vi "IRMouseAttempt.vi"() -> ()   [LabVIEW 2009]
uses:
  wiimotestate.ctl
  wiimoteState(IR).ctl
  C:/Documents and Settings/pbooth/My Documents/labWOOOO/WiimoteLib.dll
  User32.dll
panel:
  out "IR Camera Targets":picture
  out "Cluster":cluster{"Wiimote State":T1, "IRState":T2} {"IRState"."Mode" items=["Off"=0, "Basic"=1, "Extended"=3, "Full"=5]}
  in  "stop":bool
  out "error out":errorcluster
  # "Establish a Bluetooth link with your Wiimote prior to executing this VI.\n\nRequires the Wiimote Managed Library WiimoteLib Ver 1.7\navailable from http://www.codeplex.com/WiimoteLib\nSam Shearman"
  # "Accelerometers"
  # "Buttons"
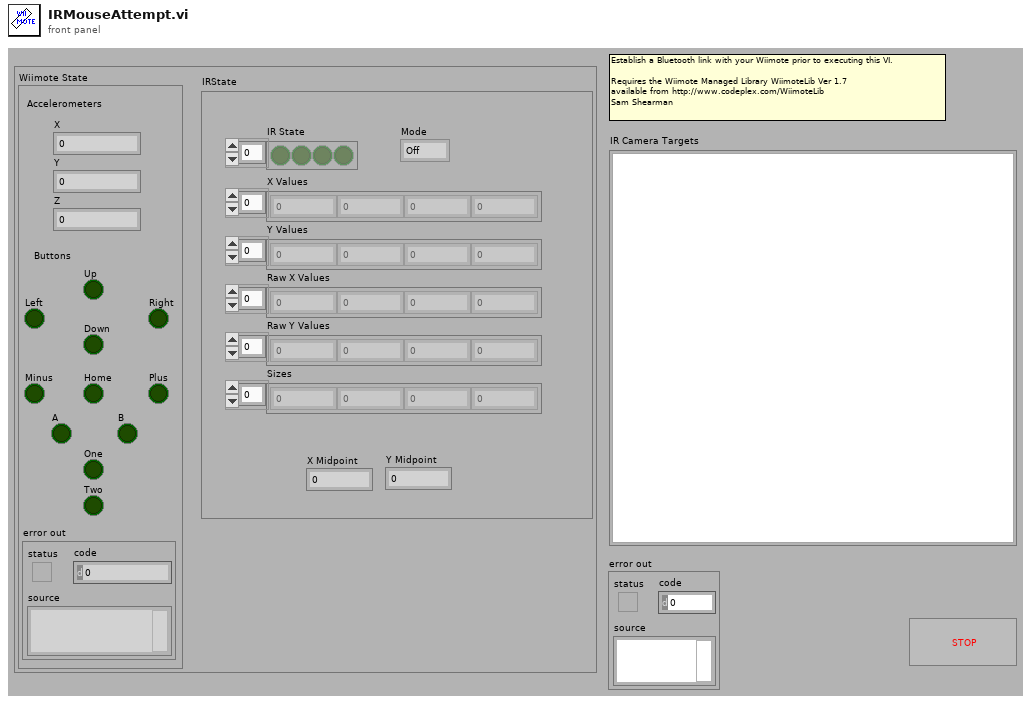
[diagram p1: front panel]
types:
  T1 = typedef "wiimotestate.ctl" = cluster{"X":sgl, "Y":sgl, "Z":sgl, "A":bool, "B":bool, "Down":bool, "Home":bool, "Left":bool, "Minus":bool, "One":bool, "Plus":bool, "Right":bool, "Two":bool, "Up":bool, "error out":errorcluster}
  T2 = typedef "wiimoteState(IR).ctl" = cluster{"Mode":u8, "IR State":bool[], "X Values":sgl[], "Y Values":sgl[], "Raw X Values":i32[], "Raw Y Values":i32[], "Sizes":i32[], "X Midpoint":sgl, "Y Midpoint":sgl}
  T3 = typedef "LVBoundsTypeDef.ctl" = cluster{"Width":u32, "Height":u32}
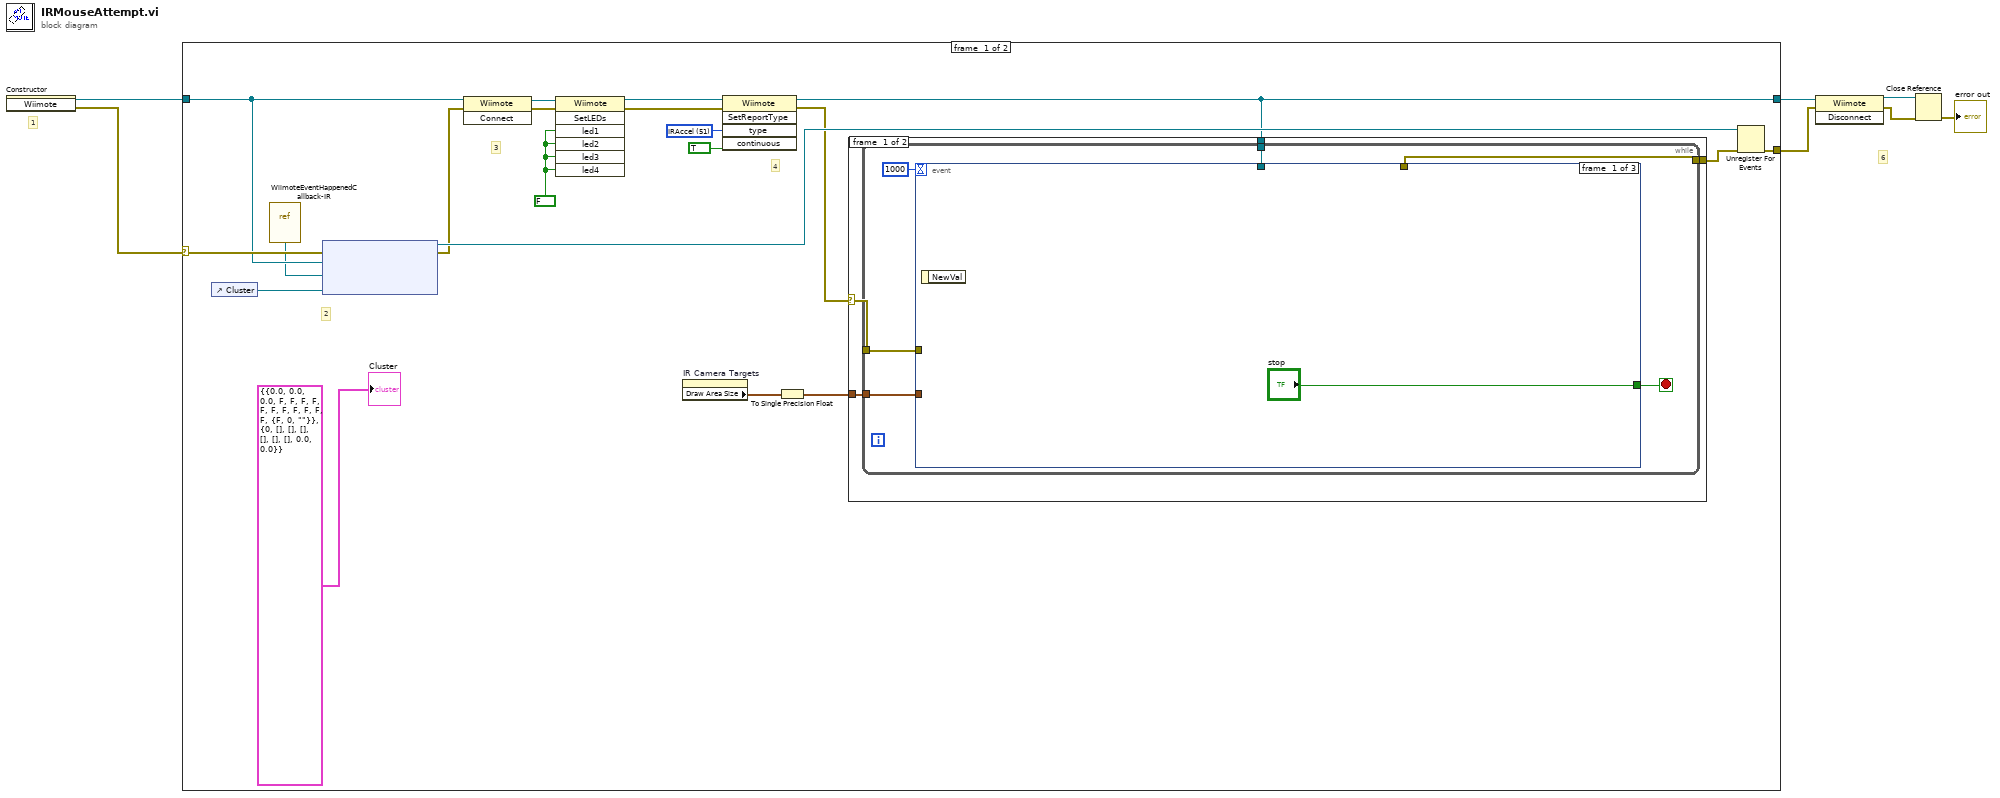
[diagram p0: block diagram]
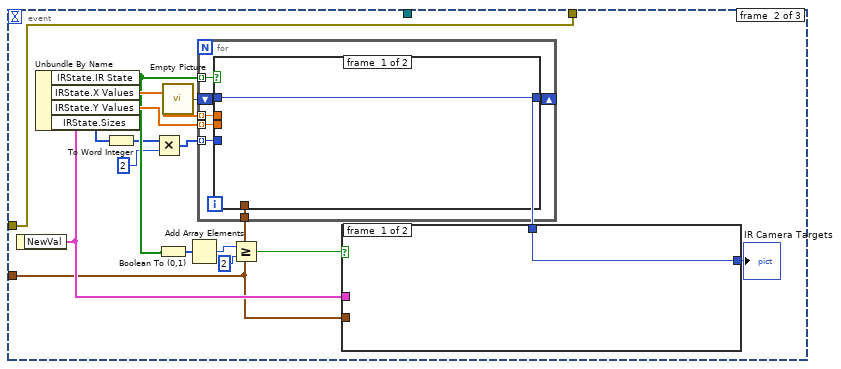
[diagram p2: hidden frame]
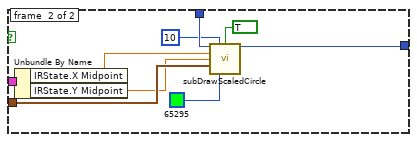
[diagram p3: hidden frame]
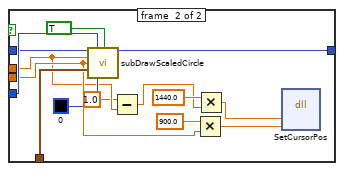
[diagram p4: hidden frame]
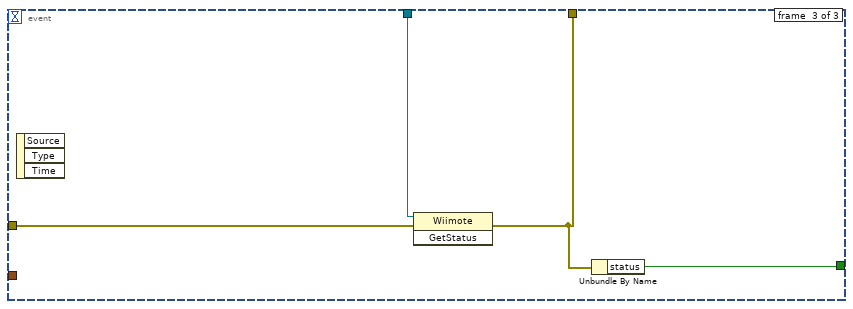
[diagram p5: hidden frame]
diagram:
  # "6"
  # "1"
  n1 = constructor class="Wiimote"() -> (reference out=w2:refnum<k24>, error out=w1:errorcluster)  [unwired: 3 in, 1 out]
  n2 = case shown="No Error" w1 {
    selector: w1 -> [w21 w94]
    tunnel: [w26 w94] -> w5
    tunnel: [w20 w93] -> w3
    tunnel: w2 -> [w10 w93]
    frame #0 {
      w23 = u8 51 items=["Status"=32, "ReadData"=33, "Buttons"=48, "ButtonsAccel"=49, "IRAccel"=51, "ButtonsExtension"=52, "ExtensionAccel"=53, "IRExtensionAccel"=55] ("type")
      w17 = FALSE ("continuous")
      # "2"
      # "4"
      # "3"
      n3 = control-ref of="Cluster"() -> (w27:refnum<vi>)
      n4 = vi-ref "WiimoteEventHappenedCallback-IR.vi"() -> ("vi reference"=w8:refnum<vi>)
      n5 = node(w21, w10, w8, w27) -> (w24:refnum<k27>, w19:errorcluster)  [unwired: 1 in]
      n6 = invoke class="Wiimote" method="Connect"(reference=w10, error in=w19) -> (reference out=w18:refnum<k24>, error out=w15:errorcluster)  [unwired: 1 in, 1 out]
      n7 = invoke class="Wiimote" method="SetLEDs"(reference=w18, error in=w15, "led1"=w17, "led2"=w17, "led3"=w17, "led4"=w17) -> (reference out=w16:refnum<k24>, error out=w14:errorcluster)  [unwired: 1 in, 5 out]
      n8 = property on="IR Camera Targets" class="Pict"() -> ("Draw Area Size"=w12:T3)  [unwired: 2 in, 2 out]
      n9 = invoke class="Wiimote" method="SetReportType"(reference=w16, error in=w14, "type"=w23, "continuous"=TRUE) -> (reference out=w20:refnum<k24>, error out=w11:errorcluster)  [unwired: 1 in, 3 out]
      n10 = To Single Precision Float(number=w12) -> (single precision float=w13:cluster{"Width":sgl, "Height":sgl})
      n11 = case shown="No Error" w11 {
        selector: w11 -> [w28 w92]
        tunnel: [w31 w92] -> w25
        tunnel: w20 -> [w30 _]
        tunnel: w13 -> [w29 _]
        frame #0 {
          n12 = while {
            tunnel: [w33] -> w31
            tunnel: w28 -> [w36]
            tunnel: w30 -> [w35]
            tunnel: w29 -> [w32]
            stop <- w37 stop-if-true
            n13 = event shown="[1] \"Cluster\": Value Change" {
              selector: _ -> [_ _ _]
              dyn-events: _ -> [_ _ _]
              timeout: 1000 -> [_ _ _]
              tunnel: ["stop" _ w89] -> w37
              tunnel: w36 -> [_ w48 w91]
              tunnel: w35 -> [_ _ w90]
              tunnel: [_ w48 w88] -> w33
              tunnel: w32 -> [_ w49 _]
              event #0 {
                n14 = event-data() -> ()  [unwired: 2 out]
              }
              event #1 {
                n15 = event-data() -> ("NewVal"=w52:cluster{"Wiimote State":T1, "IRState":T2})  [unwired: 1 out]
                n16 = Unbundle By Name(w52) -> ("IRState.IR State"=w47:bool[], "IRState.X Values"=w53:sgl[], "IRState.Y Values"=w54:sgl[], "IRState.Sizes"=w42:i32[])
                n17 = To Word Integer(number=w42) -> (16bit integer=w39:i16[])
                n18 = Multiply(x=w39, y=i16 2) -> (x*y=w41:i16[])
                n19 = Boolean To (0,1)(Boolean=w47) -> (0, 1=w46:i16[])
                n20 = call "Empty Picture"() -> ("empty picture"=w55:picture)
                n21 = Add Array Elements(numeric array=w46) -> (sum=w44:i16)
                n22 = for {
                  shift-right: [w71] -> w50
                  shift-left: w55 -> [w72]
                  tunnel: w41 -> [w70] mode=indexing
                  tunnel: w53 -> [w69] mode=indexing
                  tunnel: w54 -> [w68] mode=indexing
                  tunnel: w49 -> [w67]
                  tunnel: w47 -> [w66] mode=indexing
                  n23 = case shown="True" w66 {
                    tunnel: w72 -> [w73 w82]
                    tunnel: [w73 w87] -> w71
                    tunnel: w70 -> [_ w83]
                    tunnel: w69 -> [_ w76]
                    tunnel: w68 -> [_ w77]
                    tunnel: w67 -> [_ w86]
                    frame #0 {
                    }
                    frame #1 {
                      n24 = call "subDrawScaledCircle.vi"("picture in"=w82, "Radius"=w83, "fill?(F)"=TRUE, "X"=w76, "Y"=w77, "Display Size"=w86, "color(black)"=u32 0) -> ("picture out"=w87:picture)  [unwired: 1 in, 7 out]
                      n25 = Subtract(x=sgl 1.0, y=w76) -> (x-y=w74:sgl)
                      n26 = Multiply(x=900.0, y=w77) -> (x*y=w78:dbl)
                      n27 = Multiply(x=1440.0, y=w74) -> (x*y=w81:dbl)
                      n28 = dll-call lib="User32.dll" fn="SetCursorPos"(w81, w78) -> ()  [unwired: 5 in, 3 out]
                    }
                  }
                }
                n29 = Greater Or Equal?(x=w44, y=i16 2) -> (x >= y?=w45:bool)
                n30 = case shown="True" w45 {
                  tunnel: w52 -> [_ w65]
                  tunnel: [w56 w62] -> w51
                  tunnel: w50 -> [w56 w63]
                  tunnel: w49 -> [_ w60]
                  frame #0 {
                  }
                  frame #1 {
                    n31 = Unbundle By Name(w65) -> ("IRState.X Midpoint"=w57:sgl, "IRState.Y Midpoint"=w58:sgl)
                    n32 = call "subDrawScaledCircle.vi"("picture in"=w63, "Radius"=i16 10, "fill?(F)"=TRUE, "X"=w57, "Y"=w58, "Display Size"=w60, "color(black)"=u32 65295) -> ("picture out"=w62:picture)  [unwired: 1 in, 7 out]
                  }
                }
                "IR Camera Targets" <- w51
              }
              event #2 {
                n33 = event-data() -> ()  [unwired: 4 out]
                n34 = invoke class="Wiimote" method="GetStatus"(reference=w90, error in=w91) -> (error out=w88:errorcluster)  [unwired: 1 in, 2 out]
                n35 = Unbundle By Name(w88) -> ("status"=w89:bool)
              }
            }
          }
        }
        frame #1 {
        }
      }
      n36 = Unregister For Events(event registration refnum=w24, error in=w25) -> (error out=w26:errorcluster)
      "Cluster" <- cluster{"Wiimote State":T1, "IRState":T2} {"Wiimote State"={"X"=0.0, "Y"=0.0, "Z"=0.0, "A"=FALSE, "B"=FALSE, "Down"=FALSE, "Home"=FALSE, "Left"=FALSE, "Minus"=FALSE, "One"=FALSE, "Plus"=FALSE, "Right"=FALSE, "Two"=FALSE, "Up"=FALSE, "error out"={"status"=FALSE, "code"=0, "source"=""}}, "IRState"={"Mode"=0, "IR State"=[], "X Values"=[], "Y Values"=[], "Raw X Values"=[], "Raw Y Values"=[], "Sizes"=[], "X Midpoint"=0.0, "Y Midpoint"=0.0}} ("Cluster")
    }
    frame #1 {
    }
  }
  n37 = invoke class="Wiimote" method="Disconnect"(reference=w3, error in=w5) -> (reference out=w7:refnum<k24>, error out=w4:errorcluster)  [unwired: 1 in, 1 out]
  n38 = Close Reference(reference=w7, error in (no error)=w4) -> (error out=→"error out":errorcluster)
